vi "Oxford visa write read.vi"(8 "error in (no error)":errorcluster, 10 "write buffer":string, 11 "VISA resource name":refnum<visa-resource-name>) -> (0 "error out":errorcluster, 2 "read buffer":string, 3 "VISA resource name out":refnum<visa-resource-name>)   [LabVIEW 2015]
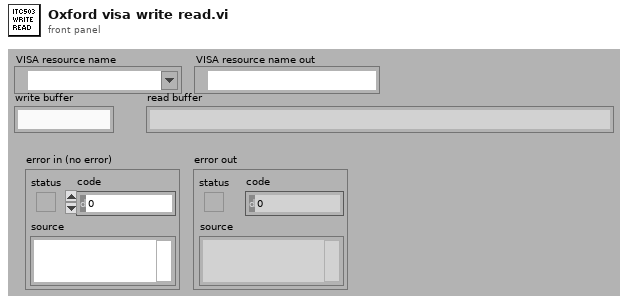
[diagram p1: front panel]
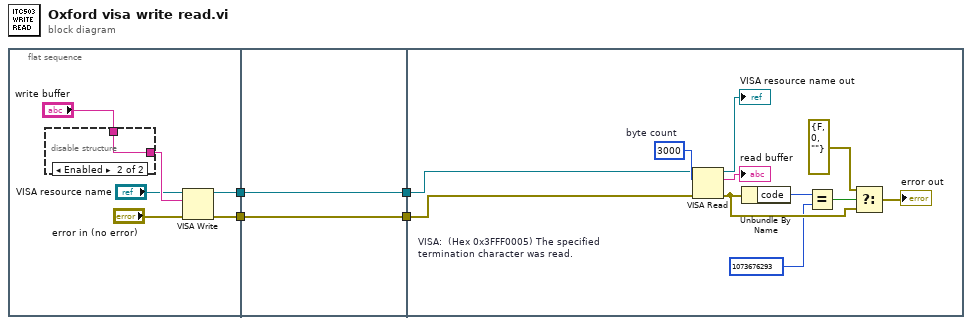
[diagram p0: block diagram]
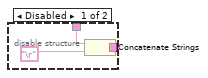
[diagram p2: hidden frame]
diagram:
  n1 = flat-sequence {
    tunnel: [w10] -> w4
    tunnel: [w9] -> w3
    tunnel: w4 -> [w16]
    tunnel: w3 -> [w15]
    tunnel: [w16] -> w2
    tunnel: [w15] -> w1
    tunnel: w2 -> [w17]
    tunnel: w1 -> [w18]
    frame #0 {
      n2 = disable-structure shown="Enabled" {
        disable-tunnel: "write buffer" -> [w13 w14]
        disable-tunnel: [w12 w14] -> w7
        frame Disabled {
          n3 = Concatenate Strings(w13, "\r") -> (w12:string)
        }
        frame Enabled {
        }
      }
      n4 = VISA Write(VISA resource name="VISA resource name", write buffer=w7, error in (no error)="error in (no error)") -> (VISA resource name out=w9:refnum<visa-resource-name>, error out=w10:errorcluster)  [unwired: 1 out]
    }
    frame #1 {
    }
    frame #2 {
      w23 = 1073676293  # VISA:  (Hex 0x3FFF0005) The specified termination character was read.
      w19 = u32 3000  # byte count
      n5 = VISA Read(VISA resource name=w18, byte count=w19, error in (no error)=w17) -> (VISA resource name out=→"VISA resource name out":refnum<visa-resource-name>, read buffer=→"read buffer":string, error out=w25:errorcluster)  [unwired: 1 out]
      n6 = Unbundle By Name(w25) -> ("code"=w22:i32)
      n7 = Equal?(x=w22, y=w23) -> (x = y?=w26:bool)
      n8 = Select(t=errorcluster {"status"=FALSE, "code"=0, "source"=""}, s=w26, f=w25) -> (s? t:f=→"error out":errorcluster)
    }
  }
